vi "Configure Arbitrary Waveform Skew.vi"(8 "error in (no error)":errorcluster, 9 "Enable Skew (T: Enable)":bool=TRUE, 10 "Skew Time (0 s)":i32, 11 "VISA resource name":refnum<visa-resource-name>) -> (0 "error out":errorcluster, 3 "VISA resource name out":refnum<visa-resource-name>)   [LabVIEW 2023, in "Keysight-33500B.lvlib"]
doc: "Configures for the skew time compensation."
uses:
  Keysight-33500B.lvlib
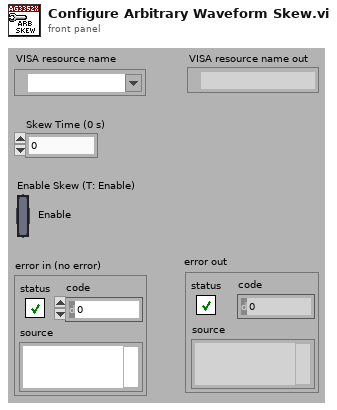
[diagram p1: front panel]
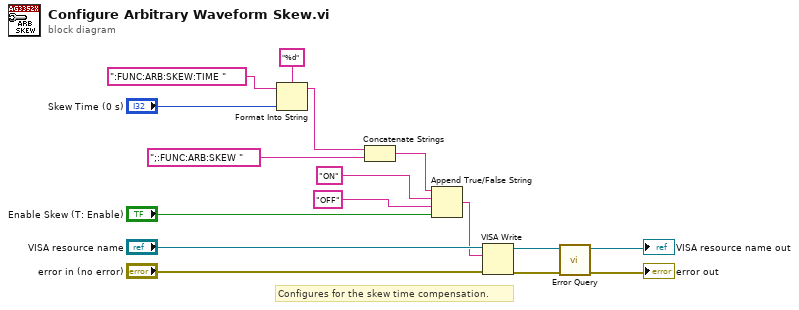
[diagram p0: block diagram]
diagram:
  # "Configures for the skew time compensation."
  n1 = Format Into String(format string="%d", initial string=":FUNC:ARB:SKEW:TIME " ("command"), "Skew Time (0 s)") -> (resulting string=w14:string)  [unwired: 1 in, 1 out]
  n2 = Concatenate Strings(w14, ";:FUNC:ARB:SKEW " ("command")) -> (w7:string)
  n3 = Append True/False String(1:"Enable Skew (T: Enable)", 2:"OFF" ("false string"), 3:"ON" ("true string"), 4:w7) -> (0:w8:string)
  n4 = VISA Write(VISA resource name="VISA resource name", write buffer=w8, error in (no error)="error in (no error)") -> (VISA resource name out=w3:refnum<visa-resource-name>, error out=w2:errorcluster)  [unwired: 1 out]
  n5 = call "Error Query.vi"("error in (no error)"=w2, "VISA resource name"=w3) -> ("error out"=→"error out":errorcluster, "VISA resource name out"=→"VISA resource name out":refnum<visa-resource-name>)  [unwired: 8 out]
